vi "TranslationalPID.vi"(7 "Translational PID Gains":T2={"proportional gain (Kc)"=1.0, "integral gain"=0.0, "derivative gain"=0.0} {"derivative gain" min=-0.1 max=0.1 step=1e-05 format="%.5f"; "integral gain" min=-10.0 max=10.0 step=1e-05 format="%.5f"; "proportional gain (Kc)" format="%.3f"}, 8 "Old Error [pixels]":dbl=-10.0, 9 "Old Integral Error [pixels*ms]":dbl=-10.0, 10 "dTime [ms]":dbl, 11 "DistanceToTarget [pixels]":T1) -> (0 "New Error [pixels]":dbl=-1.0, 1 "New Integral Error [pixel*ms]":dbl=-1.0, 3 "Translation Response":dbl=-0.022)   [LabVIEW 2015]
panel:
  # "TranslationalPID"
  # "This class generates a translational response to the movement of the tracking target withing the camera's FOV.  Essentially, it uses the Y Distance to target as the error and puts that error throgh a PID response calculation"
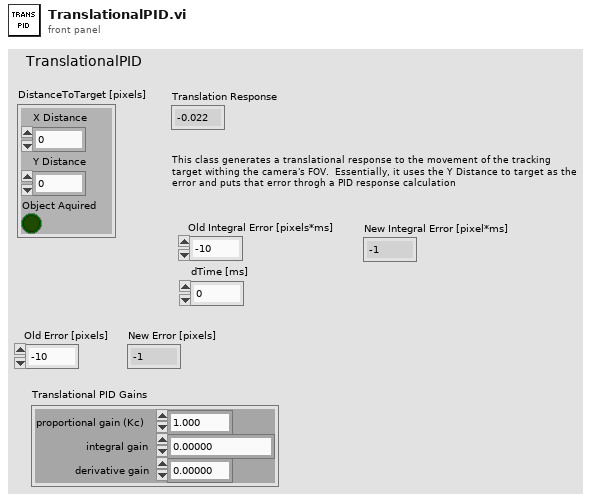
[diagram p1: front panel]
types:
  T1 = cluster{"X Distance":i32, "Y Distance":i32, "Object Aquired":bool}
  T2 = cluster{"proportional gain (Kc)":dbl, "integral gain":dbl, "derivative gain":dbl}
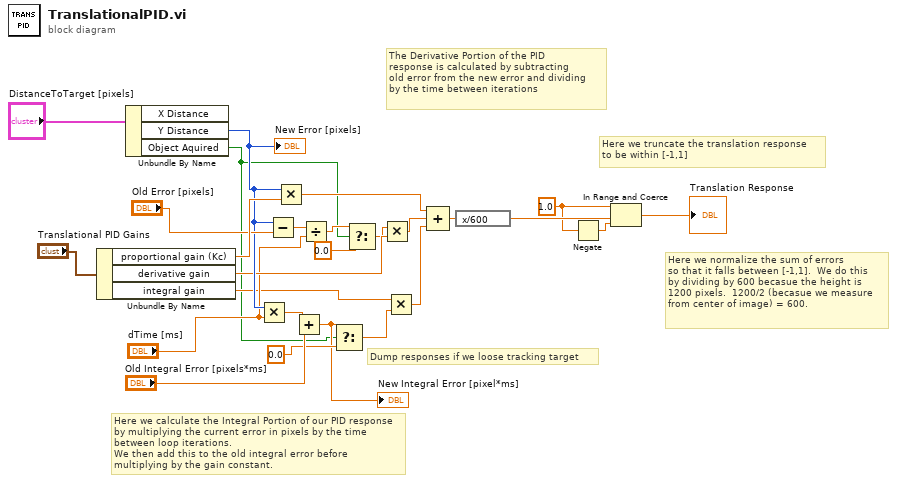
[diagram p0: block diagram]
diagram:
  w10 = 1.0 ("upper limit")
  # "Dump responses if we loose tracking target"
  # "Here we truncate the translation response \nto be within [-1,1]"
  # "The Derivative Portion of the PID\nresponse is calculated by subtracting \nold error from the new error and dividing\nby the time between iterations"
  # "Here we calculate the Integral Portion of our PID response by multiplying the current error in pixels by the time between loop iterations.\nWe then add this to the old integral error before multiplying by the gain constant."
  # "Here we normalize the sum of errors\nso that it falls between [-1,1].  We do this \nby dividing by 600 becasue the height is \n1200 pixels.  1200/2 (becasue we measure \nfrom center of image) = 600."
  n1 = Unbundle By Name("Translational PID Gains") -> ("proportional gain (Kc)"=w25:dbl, "derivative gain"=w19:dbl, "integral gain"=w12:dbl)
  n2 = Unbundle By Name("DistanceToTarget [pixels]") -> ("Y Distance"=w20:i32, "Object Aquired"=w2:bool)  [unwired: 1 out]
  "New Error [pixels]" <- w20
  n3 = Multiply(x=w20, y="dTime [ms]") -> (x*y=w18:dbl)
  n4 = Subtract(x=w20, y="Old Error [pixels]") -> (x-y=w14:dbl)
  n5 = Multiply(x=w20, y=w25) -> (x*y=w23:dbl)
  n6 = Add(x=w18, y="Old Integral Error [pixels*ms]") -> (x+y=w5:dbl)
  "New Integral Error [pixel*ms]" <- w5
  n7 = Divide(x=w14, y="dTime [ms]") -> (x/y=w3:dbl)
  n8 = Select(t=w5, s=w2, f=0.0) -> (s? t:f=w7:dbl)
  n9 = Select(t=w3, s=w2, f=0.0) -> (s? t:f=w4:dbl)
  n10 = Multiply(x=w4, y=w19) -> (x*y=w16:dbl)
  n11 = Multiply(x=w12, y=w7) -> (x*y=w17:dbl)
  n12 = Compound Arithmetic op=ADD(w23, w16, w17) -> (w22:dbl)
  n13 = expression code="x/600"(w22) -> (w21:dbl)
  n14 = Negate(x=w10) -> (-x=w9:dbl)
  n15 = In Range and Coerce(upper limit=w10, x=w21, lower limit=w9) -> (coerced(x)=→"Translation Response":dbl)  [unwired: 1 out]
